vi "HELP.vi"(1 "comando":string[](array[string]), 2 "descripcion":string[](array[string])) -> (0 "MENSAJE":string)   [LabVIEW 2020]
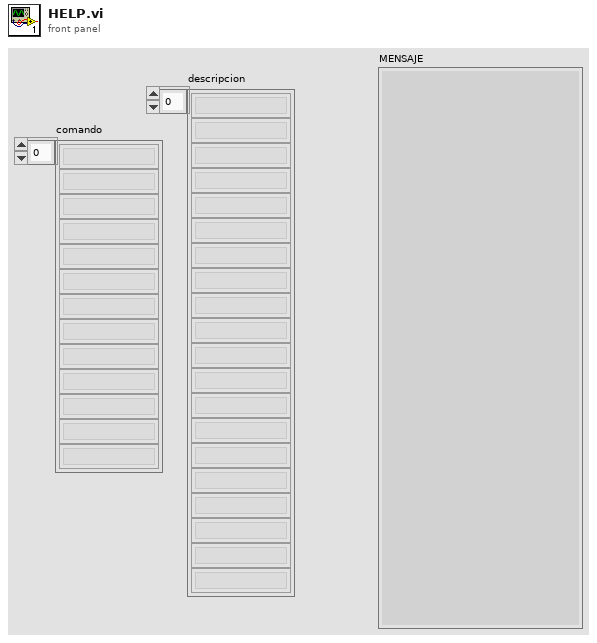
[diagram p1: front panel]
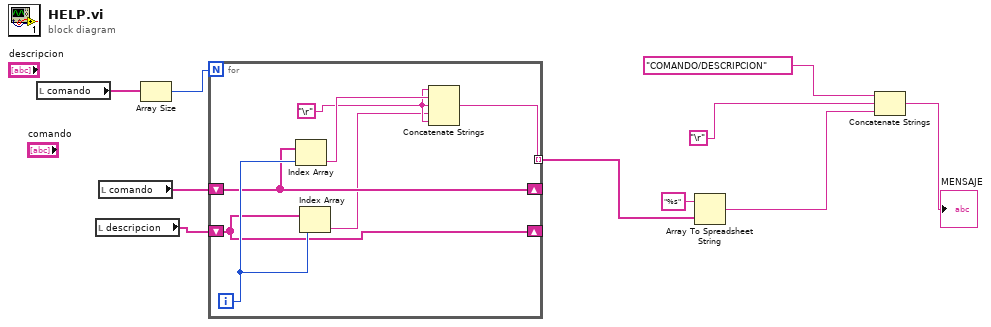
[diagram p0: block diagram]
diagram:
  n1 = local read "comando"() -> (w10:string[])
  n2 = local read "descripcion"() -> (w6:string[])
  n3 = local read "comando"() -> (w8:string[])
  n4 = Array Size(array=w10) -> (size(s)=w9:i32)
  n5 = for {
    N: w9 -> [_]
    shift-right: [w16] -> _
    shift-left: w8 -> [w16]
    shift-right: [w13] -> _
    shift-left: w6 -> [w13]
    tunnel: [w15] -> w5 mode=indexing
    i -> [w17]
    w12 = "\r"
    n6 = Index Array(array=w16, index=w17) -> (element=w14:string)
    n7 = Index Array(array=w13, index=w17) -> (element=w11:string)
    n8 = Concatenate Strings(w12, w14, w12, w11, w12) -> (w15:string)
  }
  n9 = Array To Spreadsheet String(array=w5, 3:"%s" ("format string")) -> (spreadsheet string=w3:string)  [unwired: 1 in]
  n10 = Concatenate Strings("COMANDO/DESCRIPCION", "\r", w3) -> (→"MENSAJE":string)
